vi "Apply min Threshold.vi"(8 "error in":errorcluster, 10 "Min. Thresh.":sgl, 11 "Image In":T1) -> (0 "error out":errorcluster, 3 "Image Out":T1)   [LabVIEW 2020, in "POLARIS IMAQ Display.xctl"]
uses:
  POLARIS IMAQ Display.xctl
  <vilib>/vision/Image Controls.llb/IMAQ Image.ctl
  <vilib>/vision/NI_Vision_Development_Module.lvlib
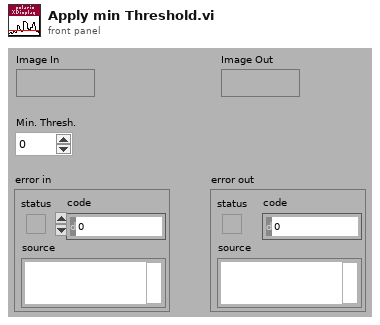
[diagram p1: front panel]
types:
  T1 = typedef "IMAQ Image.ctl" = refnum<image>
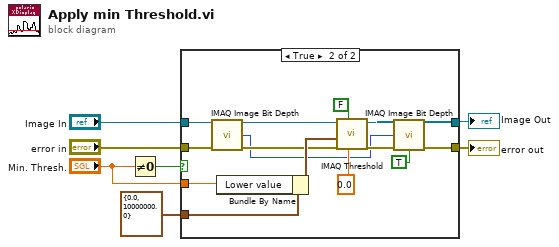
[diagram p0: block diagram]
diagram:
  n1 = Not Equal To 0?(x="Min. Thresh.") -> (x != 0?=w5:bool)
  n2 = case shown="True" w5 {
    tunnel: [w8 w24] -> w1
    tunnel: "Min. Thresh." -> [_ w23]
    tunnel: "Image In" -> [w9 w15]
    tunnel: "error in" -> [w8 w14]
    tunnel: [w9 w22] -> w3
    tunnel: cluster{"Lower value":sgl, "Upper value":sgl} {"Lower value"=0.0, "Upper value"=10000000.0} ("Tresh") -> [_ w10]
    frame False {
    }
    frame True {
      n3 = call "IMAQ Image Bit Depth"("Image"=w15, "error in (no error)"=w14) -> ("Image Out"=w11:T1, "Bit Depth"=w12:u32, "error out"=w13:errorcluster)  [unwired: 11 in]
      n4 = Bundle By Name(cluster=w10, "Lower value"=w23) -> (w19:cluster{"Lower value":sgl, "Upper value":sgl})
      n5 = call "IMAQ Threshold"("Replace Value"=sgl 0.0, "Keep/Replace Value (Replace)"=FALSE, "error in (no error)"=w13, "Range"=w19, "Image Src"=w11) -> ("error out"=w16:errorcluster, "Image Dst Out"=w17:T1)  [unwired: 5 in]
      n6 = call "IMAQ Image Bit Depth"("Image"=w17, "Bit Depth (0)"=w12, "error in (no error)"=w16, "Get/Set Bit Depth? (Set)"=TRUE) -> ("Image Out"=w22:T1, "error out"=w24:errorcluster)  [unwired: 9 in, 1 out]
    }
  }
  "Image Out" <- w3
  "error out" <- w1
